vi "Tracer_VIControlData.vi"(6 "Calltree Level":i32, 8 "Error In":errorcluster, 9 "VI Name":string) -> (0 "Error Out":errorcluster, 1 "Values":string[](array[string]))   [LabVIEW 2018, in "TracerLibrary.lvlib" / "Tracer.lvclass"]
uses:
  Tracer.lvclass
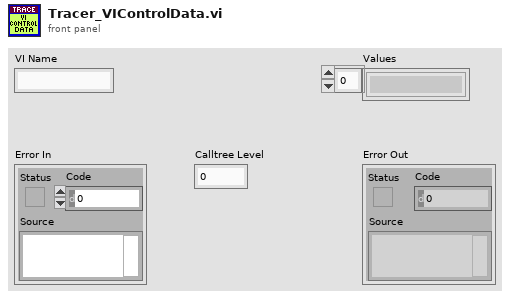
[diagram p1: front panel]
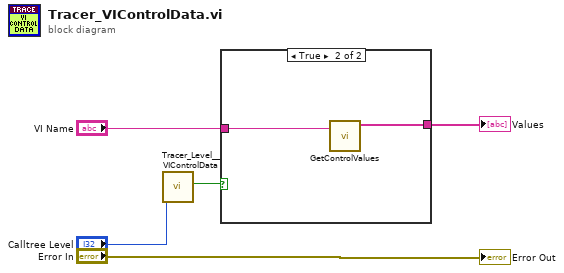
[diagram p0: block diagram]
diagram:
  n1 = call "Tracer_Level__VIControlData.vi"("Calltree Level"="Calltree Level") -> ("Trace Enabled"=w1:bool)  [unwired: 9 in, 1 out]
  n2 = case shown="True" w1 {
    tunnel: "VI Name" -> [_ w6]
    tunnel: [_ w7] -> w3
    frame False {
    }
    frame True {
      n3 = call "GetControlValues.vi"("VI Name"=w6) -> ("Values"=w7:string[])  [unwired: 10 in]
    }
  }
  "Values" <- w3
  "Error Out" <- "Error In"
